vi "testRunCalled.vi"() -> (0 "error out":errorcluster)   [LabVIEW 2019, in "TestCaseTest.lvlib"]
uses:
  TestCaseTest.lvlib
  TestCaseTestSupport/TestResultMock/TestResultMock.lvclass
  C:/Users/de200256/Code/LVUnit/TestResult/TestResult.lvclass
  TestCase/TestCase/TestCase.lvclass
  Assertion/Assertion.lvlib
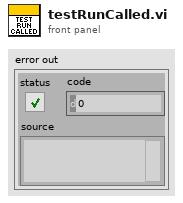
[diagram p1: front panel]
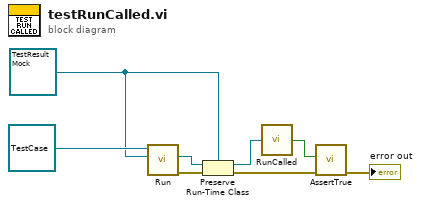
[diagram p0: block diagram]
diagram:
  w6 = refnum<class "TestResultMock.lvclass"> refnum ("TestCaseTest.lvlib:Support.lvlib:TestResultMock.lvclass")
  n1 = call-dynamic "Run.vi"("TestResult"=w6, "TestCase in"=refnum<class "TestCase.lvclass"> refnum ("TestCase.lvclass")) -> ("error out"=w3:errorcluster, "TestResult out"=w7:refnum<class "TestResult.lvclass">)  [unwired: 7 in, 1 out]
  n2 = Preserve Run-Time Class(object in=w7, error in=w3, 2:w6) -> (object out=w5:refnum<class "TestResultMock.lvclass">, error out=w2:errorcluster)
  n3 = call "RunCalled.vi"("TestResultMock In"=w5) -> ("Run Called"=w4:bool)
  n4 = call "AssertTrue.vi"("error in (no error)"=w2, "Condition"=w4) -> ("error out"=→"error out":errorcluster)  [unwired: 9 in]
